vi "Update Waveform Table.vi"(8 "error in (no error)":errorcluster, 10 "Table":i16[](array[numeric]), 11 "Data in":T1) -> (0 "error out":errorcluster)   [LabVIEW 2017, in "Test Bench.lvlib"]
uses:
  Test Bench.lvlib
  Scan Engine Variables.ctl
  <instrlib>/_niInstr/FIFO Register Bus/v1/Host/niInstr FIFO Register Bus v1 Host.lvclass
  C:/Program Files (x86)/National Instruments/LabVIEW 2017/instr.lib/_niInstr/Instruction Framework/v1/Host/Instruction Target/niInstr Instruction Target v1 Host.lvclass
  <instrlib>/_niInstr/Instruction Framework/v1/Host/Instruction Framework Context/niInstr Instruction Framework Context v1 Host.lvclass
  <instrlib>/_niInstr/Instruction Framework/v1/Host/Instruction Target/Public/Uncontextualized Write Instruction.ctl
  <instrlib>/_niInstr/Instruction Framework/v1/Host/Instruction Target/niInstr Instruction Target v1 Host.lvclass
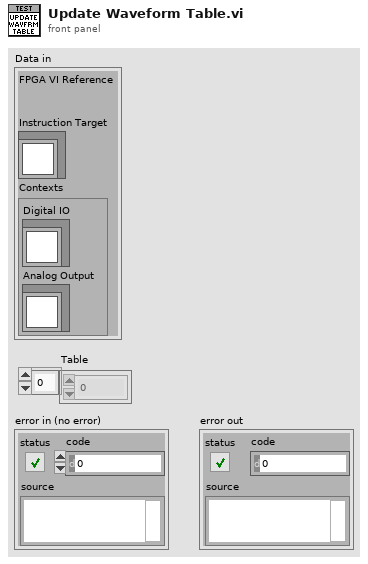
[diagram p1: front panel]
types:
  T1 = typedef "Test Bench.lvlib/Scan Engine Variables.ctl" = cluster{"FPGA VI Reference":refnum<k20>, "Instruction Target":refnum<class "niInstr FIFO Register Bus v1 Host.lvclass">, "Contexts":cluster{"Digital IO":refnum<class "niInstr Instruction Framework Context v1 Host.lvclass">, "Analog Output":refnum<class "niInstr Instruction Framework Context v1 Host.lvclass">}}
  T2 = typedef "niInstr Instruction Target v1 Host.lvclass/Uncontextualized Write Instruction.ctl" = cluster{"address":u64, "data":u64}
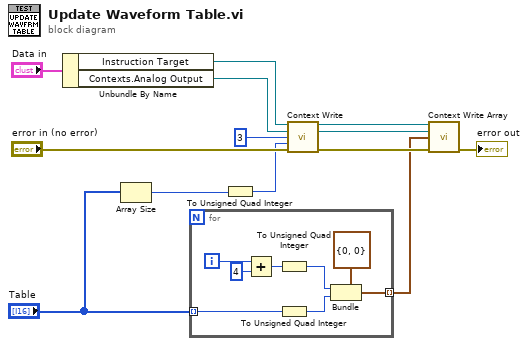
[diagram p0: block diagram]
diagram:
  n1 = Unbundle By Name("Data in") -> ("Instruction Target"=w11:refnum<class "niInstr FIFO Register Bus v1 Host.lvclass">, "Contexts.Analog Output"=w10:refnum<class "niInstr Instruction Framework Context v1 Host.lvclass">)
  n2 = Array Size(array="Table") -> (size(s)=w4:i32)
  n3 = for {
    tunnel: "Table" -> [w18] mode=indexing
    tunnel: [w15] -> w1 mode=indexing
    i -> [w21]
    n4 = Add(x=w21, y=4) -> (x+y=w19:i32)
    n5 = To Unsigned Quad Integer(1:w19) -> (0:w16:u64)
    n6 = To Unsigned Quad Integer(1:w18) -> (0:w17:u64)
    n7 = Bundle(cluster=T2 {"address"=0, "data"=0} ("uncontextualized write instruction"), "address"=w16, "data"=w17) -> (w15:T2)
  }
  n8 = To Unsigned Quad Integer(1:w4) -> (0:w3:u64)
  n9 = call <instrlib>:"Context Write.vi"("instruction target in"=w11, "context in"=w10, "address"=u64 3, "data"=w3, "error in"="error in (no error)") -> ("instruction target out"=w8:refnum<class "niInstr FIFO Register Bus v1 Host.lvclass">, "context out"=w5:refnum<class "niInstr Instruction Framework Context v1 Host.lvclass">, "error out"=w7:errorcluster)  [unwired: 8 in]
  n10 = call <instrlib>:"Context Write Array.vi"("instruction target in"=w8, "context in"=w5, "write instructions"=w1, "error in"=w7) -> ("error out"=→"error out":errorcluster)  [unwired: 9 in, 2 out]
